vi "Teleop.vi"(10 "Match Info":T1={"Autonomous Elapsed Seconds"=0.0, "TeleOp Elapsed Seconds"=0.0, "Disabled Elapsed Seconds"=0.0, "Visited Autonomous"=FALSE, "Visited TeleOp"=FALSE, "Visited Disabled"=FALSE, "Autonomous Settings"={"Autonomous Style"=enum."Independent", "VI Refnum"=refnum}}, 11 "Call Context":T2) -> ()   [LabVIEW 2017]
doc: "This VI is called for each TeleOp packet received from the DS where the robot is not disabled. It is often used to read from the joysticks and update I/O or to update setpoints for timed control loops. It should complete and return within 20 milliseconds or it may miss DS packets."
uses:
  <vilib>/Rock Robotics/WPI/DriverStation/WPI_DriverStationDerivedRobotMode.ctl
  <vilib>/Rock Robotics/WPI/DriverStation/WPI_DriverStationMatch Info.ctl
  <vilib>/Rock Robotics/WPI/Solenoid/WPI_SolenoidValue.ctl
  <vilib>/Rock Robotics/WPI/Utilities/WPI_GetSetVariantRefNum.vi
  <vilib>/Rock Robotics/Network Tables/NT Write Boolean Array.vi
  <vilib>/Rock Robotics/Network Tables/NT Write Numeric Array.vi
  <vilib>/Rock Robotics/Network Tables/NT Read Boolean.vi
  <vilib>/Rock Robotics/Network Tables/NT Read Number.vi
  <vilib>/Rock Robotics/WPI/Solenoid/WPI_SolenoidSetEnum.vi
panel:
  out "Sample Slider 0":dbl(slide) scale=0.0..5.0
  out "Sample Boolean 1":bool
  out "Sample Boolean 0":bool
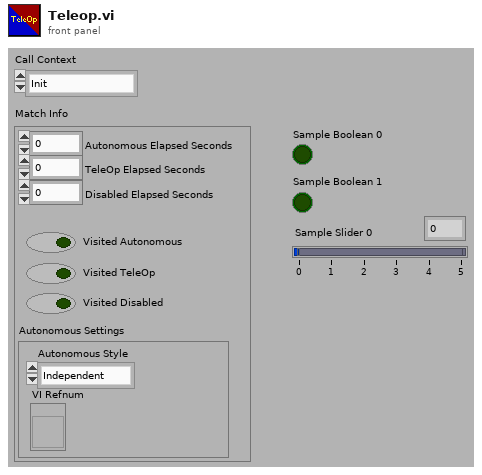
[diagram p1: front panel]
types:
  T1 = typedef "WPI_DriverStationMatch Info.ctl" = cluster{"Autonomous Elapsed Seconds":dbl, "TeleOp Elapsed Seconds":dbl, "Disabled Elapsed Seconds":dbl, "Visited Autonomous":bool, "Visited TeleOp":bool, "Visited Disabled":bool, "Autonomous Settings":cluster{"Autonomous Style":enum16{"Iterative", "Independent"}, "VI Refnum":refnum<vi>}}
  T2 = typedef "WPI_DriverStationDerivedRobotMode.ctl" = enum16{"Init", "Execute", "Stop"}
  T3 = typedef "WPI_SolenoidValue.ctl" = enum16{"Off", "On", "Forward", "Reverse"}
  T4 = typedef "WPI_CompressorDevRef.ctl" = cluster{"DevStatus":errorcluster, "Pneumatics Control Module":u8}
  T5 = typedef "WPI_RobotDriveDevRef.ctl" = cluster{"DevStatus":errorcluster, "Motors[]":T6[], "Square Inputs":bool, "Max Output":dbl}
  T6 = typedef "WPI_MotorControlDeviceRef.ctl" = cluster{"DeviceStatus":errorcluster, "Type":T7, "PWM":cluster{"PWM Channel":T8, "DeadBand":T9}, "CAN":cluster{"Device Number":u8, "SetOutput VI Ref":variant, "GetOutput VI Ref":variant, "Enable VI Ref":variant, "Disable VI Ref":variant, "Data":variant}, "Invert":bool, "DIO PWM":cluster{"PWM \"Enable\" Channel":T8, "DIOChannel":T10, "PWM Rate":dbl}}
  T7 = typedef "WPI_MotorControlType.ctl" = enum16{"PWM", "CAN", "DIO PWM"}
  T8 = typedef "FPGA_DIOPWMChannel.ctl" = enum8{"PWM 0", "PWM 1", "PWM 2", "PWM 3", "PWM 4", "PWM 5", "PWM 6", "PWM 7", "PWM 8", "PWM 9", "PWM MXP 0", "PWM MXP 1", "PWM MXP 2", "PWM MXP 3", "PWM MXP 4", "PWM MXP 5", "PWM MXP 6", "PWM MXP 7", "PWM MXP 8", "PWM MXP 9", "Invalid"}
  T9 = typedef "WPI_PWMDeadband.ctl" = cluster{"Name":string, "maxPositivePwm":i32, "minPositivePwm":i32, "centerPwm":i32, "maxNegativePwm":i32, "minNegativePwm":i32, "angularRange":u16}
  T10 = typedef "FPGA_DIOChannel.ctl" = enum8{"DIO 0", "DIO 1", "DIO 2", "DIO 3", "DIO 4", "DIO 5", "DIO 6", "DIO 7", "DIO 8", "DIO 9", "DIO MXP 0", "DIO MXP 1", "DIO MXP 2", "DIO MXP 3", "DIO MXP 4", "DIO MXP 5", "DIO MXP 6", "DIO MXP 7", "DIO MXP 8", "DIO MXP 9", "DIO MXP 10", "DIO MXP 11", "DIO MXP 12", "DIO MXP 13", "DIO MXP 14", "DIO MXP 15", "SPI Port CS1", "SPI Port CS2", "SPI Port CS3", "SPI Port MISO", "SPI Port MOSI", "Invalid"}
  T11 = typedef "WPI_JoystickDevRef.ctl" = cluster{"Device":T12}
  T12 = typedef "WPI_JoystickDeviceEnum.ctl" = enum16{"USB 0", "USB 1", "USB 2", "USB 3", "USB 4", "USB 5"}
  T13 = typedef "WPI_SolenoidDevRef.ctl" = cluster{"DevStatus":errorcluster, "Pneumatics Control Module":u8, "Forward Solenoid Channel":T14, "Reverse Solenoid Channel":T14}
  T14 = typedef "WPI_SolenoidChannel.ctl" = enum8{"Solenoid 0", "Solenoid 1", "Solenoid 2", "Solenoid 3", "Solenoid 4", "Solenoid 5", "Solenoid 6", "Solenoid 7", "Invalid"}
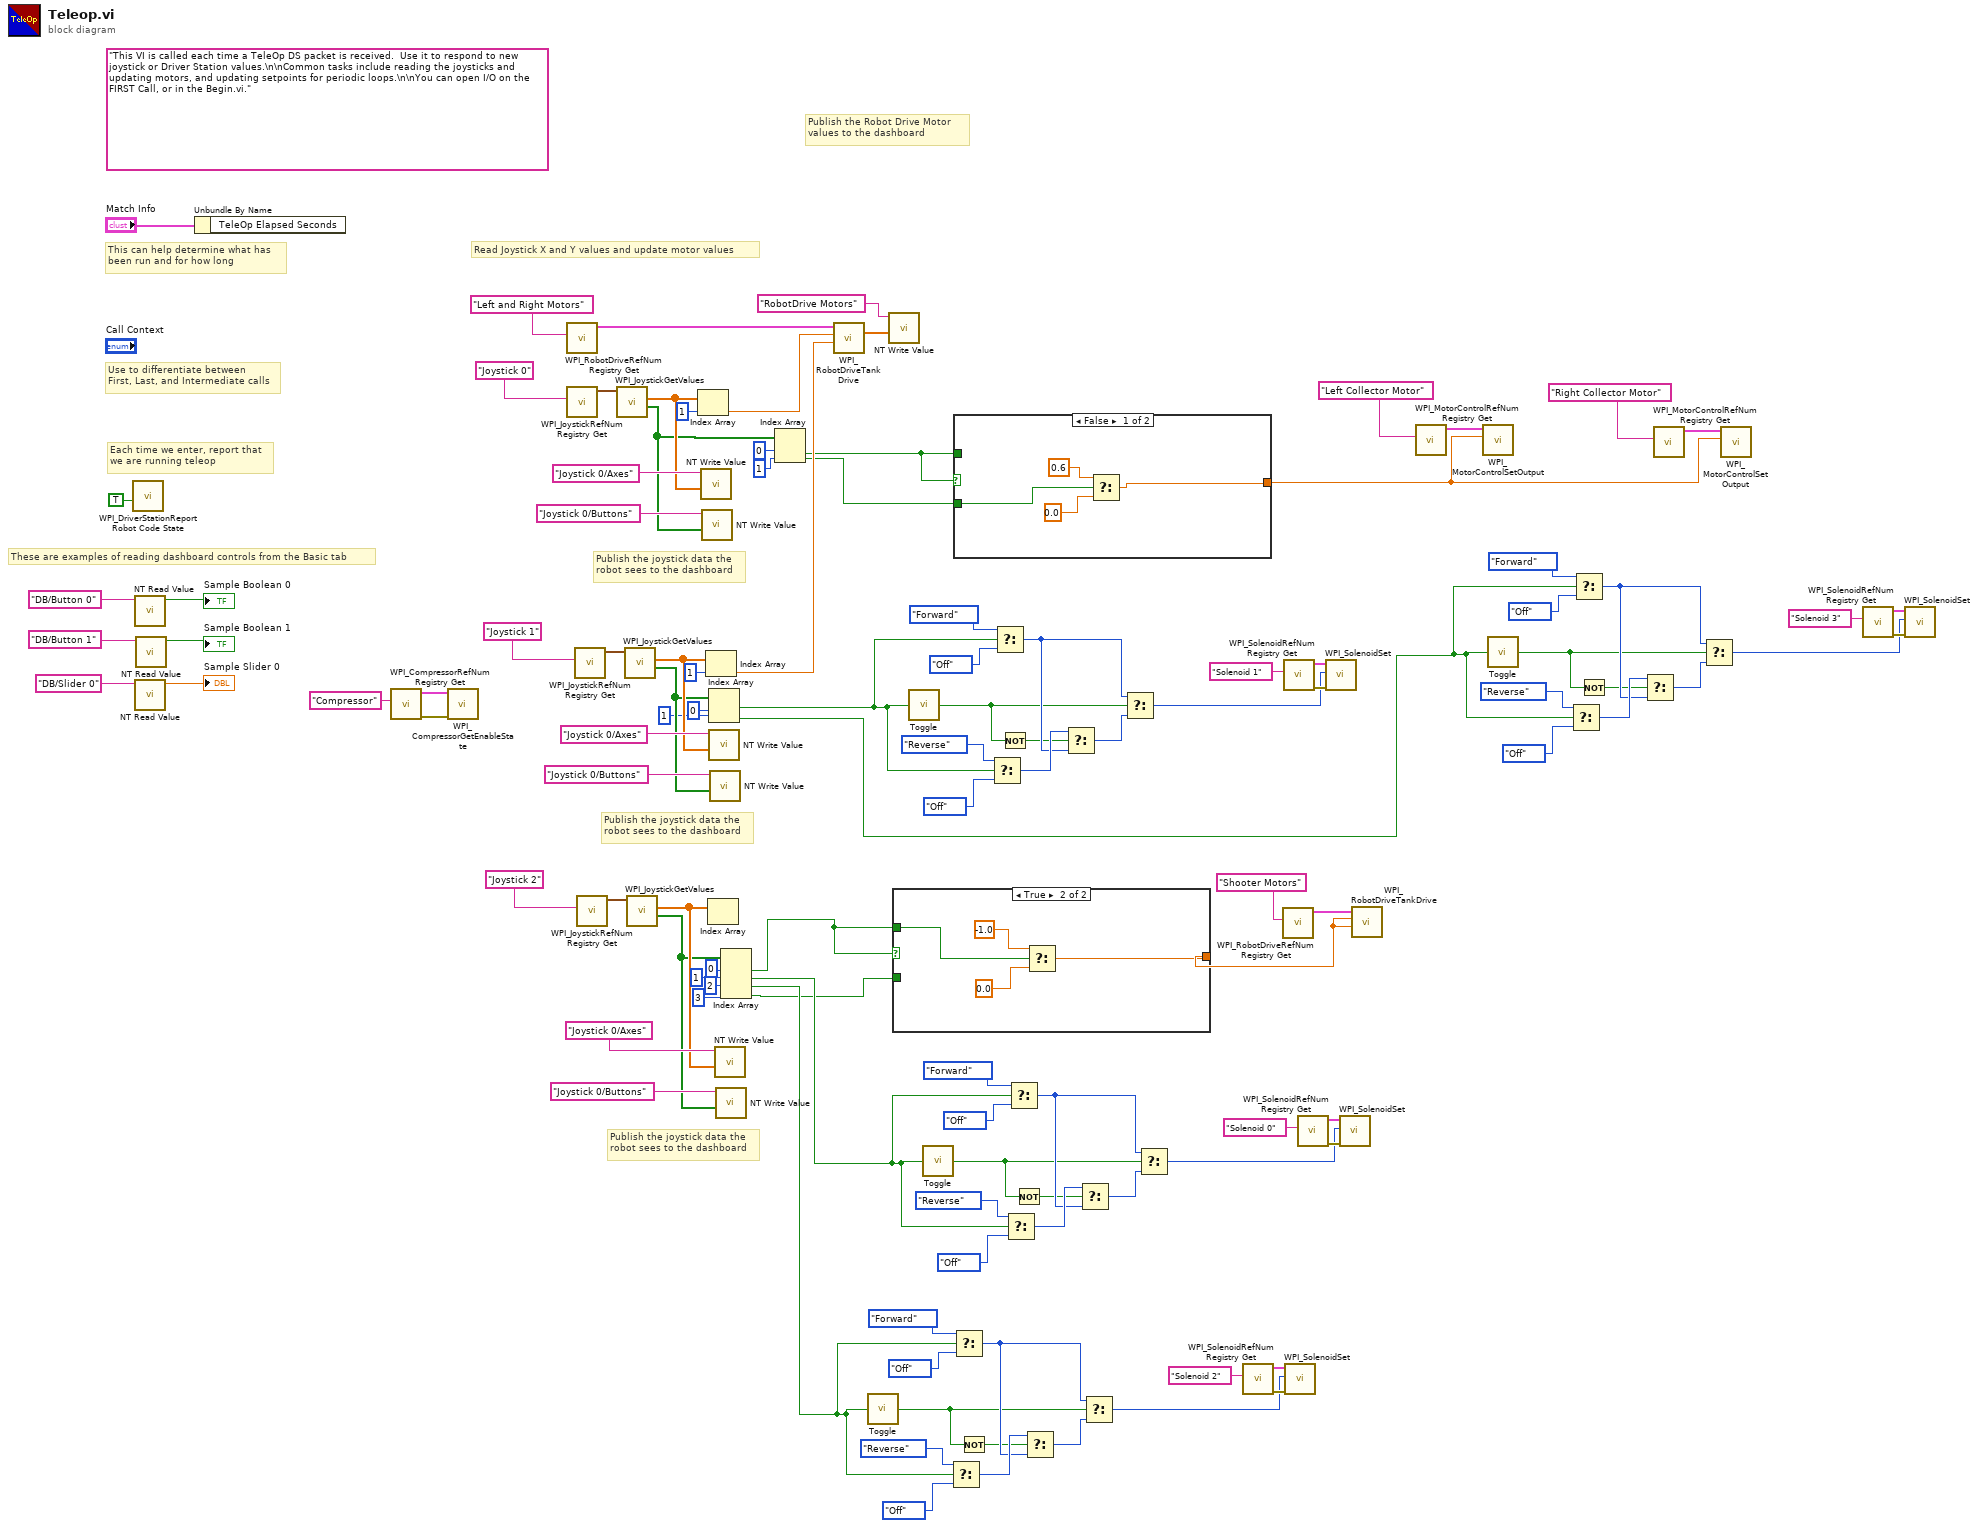
[diagram p0: block diagram]
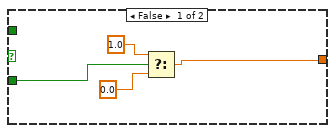
[diagram p2: hidden frame]
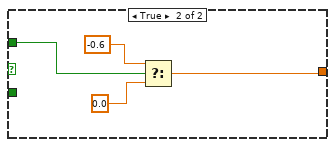
[diagram p3: hidden frame]
diagram:
  (unwired) "This VI is called each time a TeleOp DS packet is received.  Use it to respond to new joystick or Driver Station values.\n\nCommon tasks include reading the joysticks and updating motors, and updating setpoints for periodic loops.\n\nYou can open I/O on the FIRST Call, or in the Begin.vi."
  # "Publish the joystick data the\nrobot sees to the dashboard"
  # "Publish the joystick data the\nrobot sees to the dashboard"
  # "These are examples of reading dashboard controls from the Basic tab"
  # "Publish the Robot Drive Motor\nvalues to the dashboard"
  # "Publish the joystick data the\nrobot sees to the dashboard"
  # "Each time we enter, report that\nwe are running teleop"
  # "Use to differentiate between\nFirst, Last, and Intermediate calls"
  # "This can help determine what has\nbeen run and for how long"
  # "Read Joystick X and Y values and update motor values"
  n1 = call <vilib>:"WPI_DriverStationReport Robot Code State.vi"("TeleOp"=TRUE ("Autonomous")) -> ()  [unwired: 10 in, 1 out]
  n2 = call-poly <vilib>:"NT Read Value.vi"("Name"="DB/Button 0" ("refnum name")) -> ("Boolean"=→"Sample Boolean 0":bool)  [unwired: 9 in, 1 out]
  n3 = call-poly <vilib>:"NT Read Value.vi"("Name"="DB/Slider 0" ("refnum name")) -> ("Numeric"=→"Sample Slider 0":dbl)  [unwired: 9 in, 1 out]
  n4 = call-poly <vilib>:"NT Read Value.vi"("Name"="DB/Button 1" ("refnum name")) -> ("Boolean"=→"Sample Boolean 1":bool)  [unwired: 9 in, 1 out]
  n5 = Unbundle By Name("Match Info") -> ()  [unwired: 1 out]
  n6 = call <vilib>:"WPI_CompressorRefNum Registry Get.vi"("refnum name"="Compressor") -> ("error out"=w63:errorcluster, "CompressorDevRef"=w64:T4)  [unwired: 9 in]
  n7 = call <vilib>:"WPI_CompressorGetEnableState.vi"("error in (no error)"=w63, "CompressorDevRef"=w64) -> ()  [unwired: 6 in, 4 out]
  n8 = call <vilib>:"WPI_RobotDriveRefNum Registry Get.vi"("refnum name"="Left and Right Motors") -> ("RobotDriveDevRef"=w111:T5)  [unwired: 1 in, 9 out]
  n9 = call <vilib>:"WPI_JoystickRefNum Registry Get.vi"("refnum name"="Joystick 0") -> ("JoystickDevRef"=w109:T11)  [unwired: 1 in, 9 out]
  n10 = call <vilib>:"WPI_JoystickRefNum Registry Get.vi"("refnum name"="Joystick 1") -> ("JoystickDevRef"=w95:T11)  [unwired: 1 in, 9 out]
  n11 = call <vilib>:"WPI_JoystickRefNum Registry Get.vi"("refnum name"="Joystick 2") -> ("JoystickDevRef"=w90:T11)  [unwired: 1 in, 9 out]
  n12 = call <vilib>:"WPI_JoystickGetValues.vi"("JoystickDevRef"=w109) -> ("Buttons"=w79:bool[], "Axes"=w105:dbl[])  [unwired: 6 in, 3 out]
  n13 = call <vilib>:"WPI_JoystickGetValues.vi"("JoystickDevRef"=w95) -> ("Buttons"=w62:bool[], "Axes"=w92:dbl[])  [unwired: 6 in, 3 out]
  n14 = call <vilib>:"WPI_JoystickGetValues.vi"("JoystickDevRef"=w90) -> ("Buttons"=w84:bool[], "Axes"=w87:dbl[])  [unwired: 6 in, 3 out]
  n15 = Index Array(array=w105, index=1) -> (element=w81:dbl)
  n16 = call-poly <vilib>:"NT Write Value.vi"("Numeric Array"=w105, "Name"="Joystick 0/Axes") -> ()  [unwired: 9 in, 1 out]
  n17 = call-poly <vilib>:"NT Write Value.vi"("Boolean Array"=w79, "Name"="Joystick 0/Buttons") -> ()  [unwired: 9 in, 1 out]
  n18 = Index Array(array=w92, index=1) -> (element=w80:dbl)
  n19 = Index Array(array=w87) -> ()  [unwired: 1 in, 1 out]
  n20 = Index Array(array=w62, index #1=0 ("index"), index #2=1 ("index")) -> (element #1=w47:bool, element #2=w16:bool)
  n21 = call-poly <vilib>:"NT Write Value.vi"("Numeric Array"=w92, "Name"="Joystick 0/Axes") -> ()  [unwired: 9 in, 1 out]
  n22 = call-poly <vilib>:"NT Write Value.vi"("Boolean Array"=w62, "Name"="Joystick 0/Buttons") -> ()  [unwired: 9 in, 1 out]
  n23 = call-poly <vilib>:"NT Write Value.vi"("Numeric Array"=w87, "Name"="Joystick 0/Axes") -> ()  [unwired: 9 in, 1 out]
  n24 = call-poly <vilib>:"NT Write Value.vi"("Boolean Array"=w84, "Name"="Joystick 0/Buttons") -> ()  [unwired: 9 in, 1 out]
  n25 = Index Array(array=w84, index #1=0 ("index"), index #2=1 ("index"), index #3=2 ("index"), index #4=3 ("index")) -> (element #1=w3:bool, element #2=w31:bool, element #3=w14:bool, element #4=w1:bool)
  n26 = Index Array(array=w79, index #1=0 ("index"), index #2=1 ("index")) -> (element #1=w5:bool, element #2=w4:bool)
  n27 = call <vilib>:"WPI_RobotDriveTankDrive.vi"("Right axis value"=w80, "Left axis value"=w81, "RobotDriveDevRef"=w111) -> ("Motor Values"=w98:dbl[])  [unwired: 6 in, 2 out]
  n28 = call "Toggle.vi"("Input"=w14) -> ("Output"=w36:bool)
  n29 = call-poly <vilib>:"NT Write Value.vi"("Numeric Array"=w98, "Name"="RobotDrive Motors") -> ()  [unwired: 9 in, 1 out]
  n30 = case shown="True" w3 {
    tunnel: w3 -> [_ w119]
    tunnel: w1 -> [w117 _]
    tunnel: [w114 w118] -> w2
    frame False {
      n31 = Select(t=1.0, s=w117, f=0.0) -> (s? t:f=w114:dbl)
    }
    frame True {
      n32 = Select(t=-1.0, s=w119, f=0.0) -> (s? t:f=w118:dbl)
    }
  }
  n33 = call "Toggle.vi"("Input"=w47) -> ("Output"=w51:bool)
  n34 = call "Toggle.vi"("Input"=w31) -> ("Output"=w68:bool)
  n35 = Select(t=WPI_SolenoidValue."Reverse" ("Value"), s=w14, f=WPI_SolenoidValue."Off") -> (s? t:f=w39:T3)
  n36 = case shown="False" w5 {
    tunnel: w5 -> [_ w127]
    tunnel: w4 -> [w125 _]
    tunnel: [w122 w126] -> w8
    frame False {
      n37 = Select(t=0.6, s=w125, f=0.0) -> (s? t:f=w122:dbl)
    }
    frame True {
      n38 = Select(t=-0.6, s=w127, f=0.0) -> (s? t:f=w126:dbl)
    }
  }
  n39 = Select(t=WPI_SolenoidValue."Forward", s=w14, f=WPI_SolenoidValue."Off" ("Value")) -> (s? t:f=w37:T3)
  n40 = Not(x=w36) -> (.not. x?=w35:bool)
  n41 = Select(t=WPI_SolenoidValue."Reverse" ("Value"), s=w47, f=WPI_SolenoidValue."Off") -> (s? t:f=w54:T3)
  n42 = Select(t=WPI_SolenoidValue."Forward", s=w47, f=WPI_SolenoidValue."Off" ("Value")) -> (s? t:f=w52:T3)
  n43 = Not(x=w51) -> (.not. x?=w50:bool)
  n44 = Select(t=WPI_SolenoidValue."Reverse" ("Value"), s=w31, f=WPI_SolenoidValue."Off") -> (s? t:f=w71:T3)
  n45 = Select(t=WPI_SolenoidValue."Forward", s=w31, f=WPI_SolenoidValue."Off" ("Value")) -> (s? t:f=w69:T3)
  n46 = Not(x=w68) -> (.not. x?=w67:bool)
  n47 = Select(t=w39, s=w35, f=w37) -> (s? t:f=w38:T3)
  n48 = Select(t=w54, s=w50, f=w52) -> (s? t:f=w53:T3)
  n49 = Select(t=w71, s=w67, f=w69) -> (s? t:f=w70:T3)
  n50 = Select(t=w37, s=w36, f=w38) -> (s? t:f=w41:T3)
  n51 = Select(t=w52, s=w51, f=w53) -> (s? t:f=w48:T3)
  n52 = Select(t=w69, s=w68, f=w70) -> (s? t:f=w73:T3)
  n53 = call <vilib>:"WPI_SolenoidRefNum Registry Get.vi"("refnum name"="Solenoid 2") -> ("error out"=w45:errorcluster, "SolenoidDevRef"=w44:T13)  [unwired: 9 in]
  n54 = call <vilib>:"WPI_RobotDriveRefNum Registry Get.vi"("refnum name"="Shooter Motors") -> ("RobotDriveDevRef"=w33:T5)  [unwired: 9 in, 1 out]
  n55 = call <vilib>:"WPI_SolenoidRefNum Registry Get.vi"("refnum name"="Solenoid 1") -> ("error out"=w59:errorcluster, "SolenoidDevRef"=w58:T13)  [unwired: 9 in]
  n56 = call-poly <vilib>:"WPI_SolenoidSet.vi"("error in (no error)"=w45, "Value"=w41, "SolenoidDevRef"=w44) -> ()  [unwired: 7 in, 2 out]
  n57 = call <vilib>:"WPI_SolenoidRefNum Registry Get.vi"("refnum name"="Solenoid 0") -> ("error out"=w77:errorcluster, "SolenoidDevRef"=w76:T13)  [unwired: 9 in]
  n58 = call-poly <vilib>:"WPI_SolenoidSet.vi"("error in (no error)"=w59, "Value"=w48, "SolenoidDevRef"=w58) -> ()  [unwired: 7 in, 2 out]
  n59 = call-poly <vilib>:"WPI_SolenoidSet.vi"("error in (no error)"=w77, "Value"=w73, "SolenoidDevRef"=w76) -> ()  [unwired: 7 in, 2 out]
  n60 = call <vilib>:"WPI_RobotDriveTankDrive.vi"("Right axis value"=w2, "Left axis value"=w2, "RobotDriveDevRef"=w33) -> ()  [unwired: 6 in, 3 out]
  n61 = call <vilib>:"WPI_MotorControlRefNum Registry Get.vi"("refnum name"="Left Collector Motor") -> ("MotorControlDevRef"=w10:T6)  [unwired: 9 in, 1 out]
  n62 = call <vilib>:"WPI_MotorControlSetOutput.vi"("Output"=w8, "MotorControlDevRef"=w10) -> ()  [unwired: 7 in, 3 out]
  n63 = call "Toggle.vi"("Input"=w16) -> ("Output"=w20:bool)
  n64 = Select(t=WPI_SolenoidValue."Reverse" ("Value"), s=w16, f=WPI_SolenoidValue."Off") -> (s? t:f=w23:T3)
  n65 = Select(t=WPI_SolenoidValue."Forward", s=w16, f=WPI_SolenoidValue."Off" ("Value")) -> (s? t:f=w21:T3)
  n66 = Not(x=w20) -> (.not. x?=w19:bool)
  n67 = Select(t=w23, s=w19, f=w21) -> (s? t:f=w22:T3)
  n68 = call <vilib>:"WPI_MotorControlRefNum Registry Get.vi"("refnum name"="Right Collector Motor") -> ("MotorControlDevRef"=w12:T6)  [unwired: 9 in, 1 out]
  n69 = Select(t=w21, s=w20, f=w22) -> (s? t:f=w17:T3)
  n70 = call <vilib>:"WPI_MotorControlSetOutput.vi"("Output"=w8, "MotorControlDevRef"=w12) -> ()  [unwired: 7 in, 3 out]
  n71 = call <vilib>:"WPI_SolenoidRefNum Registry Get.vi"("refnum name"="Solenoid 3") -> ("error out"=w28:errorcluster, "SolenoidDevRef"=w27:T13)  [unwired: 9 in]
  n72 = call-poly <vilib>:"WPI_SolenoidSet.vi"("error in (no error)"=w28, "Value"=w17, "SolenoidDevRef"=w27) -> ()  [unwired: 7 in, 2 out]
